vi "Within Degree.vi"() -> (0 "Yaw":dbl, 3 "Boolean":bool)   [LabVIEW 2014]
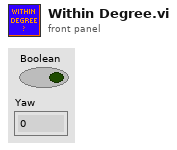
[diagram p1: front panel]
types:
  T1 = typedef "navX-MXP IMU.lvlib/navX YPRH Data.ctl" = cluster{"Yaw":dbl, "Pitch":dbl, "Roll":dbl, "Heading":dbl}
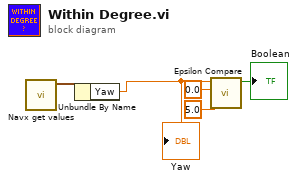
[diagram p0: block diagram]
diagram:
  n1 = call "Navx get values.vi"() -> ("YPRH"=w2:T1)  [unwired: 11 in]
  n2 = Unbundle By Name(w2) -> ("Yaw"=w1:dbl)
  "Yaw" <- w1
  n3 = call "Epsilon Compare.vi"("Epsilon"=5.0, "Value2"=0.0, "Value1"=w1) -> ("Boolean"=→"Boolean":bool)  [unwired: 8 in]
